vi "pco.camera_Avg_Example_IMAQ.vi"() -> ()   [LabVIEW 2020]
uses:
  Camera.lvclass
panel:
  out "rawImage":u16[][](array[numeric])
  out "Image":T1(plugin-control)
  in  "data_format":T2(ring)=enum."Mono16"
  out "Recorded Images":u32
  in  "Quit":bool
  in  "roiY1":u64=2 min=2 max=1040 step=1
  in  "roiX1":u64=2 min=2 max=1392 step=1
  in  "roiY0":u64=1 min=1 max=1039 step=1
  in  "roiX0":u64=1 min=1 max=1391 step=1
  out "Image Height":u64
  out "Image Width":u64
  in  "dwImgCount":u32=10 caption="Required Number of Images" max=4023
  out "Error":errorcluster {"code" format="%x"}
  # "This example shows how to continously compute and show an averaged image.\nHere the camera class is operated in sequence mode and the required number of images also defines the number of images that will be averaged\nIt is a good starting point for writing own applications.\nBut it will not be fail save, i.e. doesnt react on errors, just handles them forward to the end\n\nUsage:\nSelect your required image count you want to average over before you start the program.\nOnce started, the camera class will be initialized and image record will start automatically.\nInside the acquisition loop the program will record the image sequence.\nThen it calculates the average image and shows it.\nBy using the ROI parameters you can crop the image to select certain regions\n\nBy clicking Quit Application the record will stop and will force an exit of the camera class"
  # "pco.labview"
  # "Camera Setup"
  # "Recording Control"
  # "Parameters for image readout"
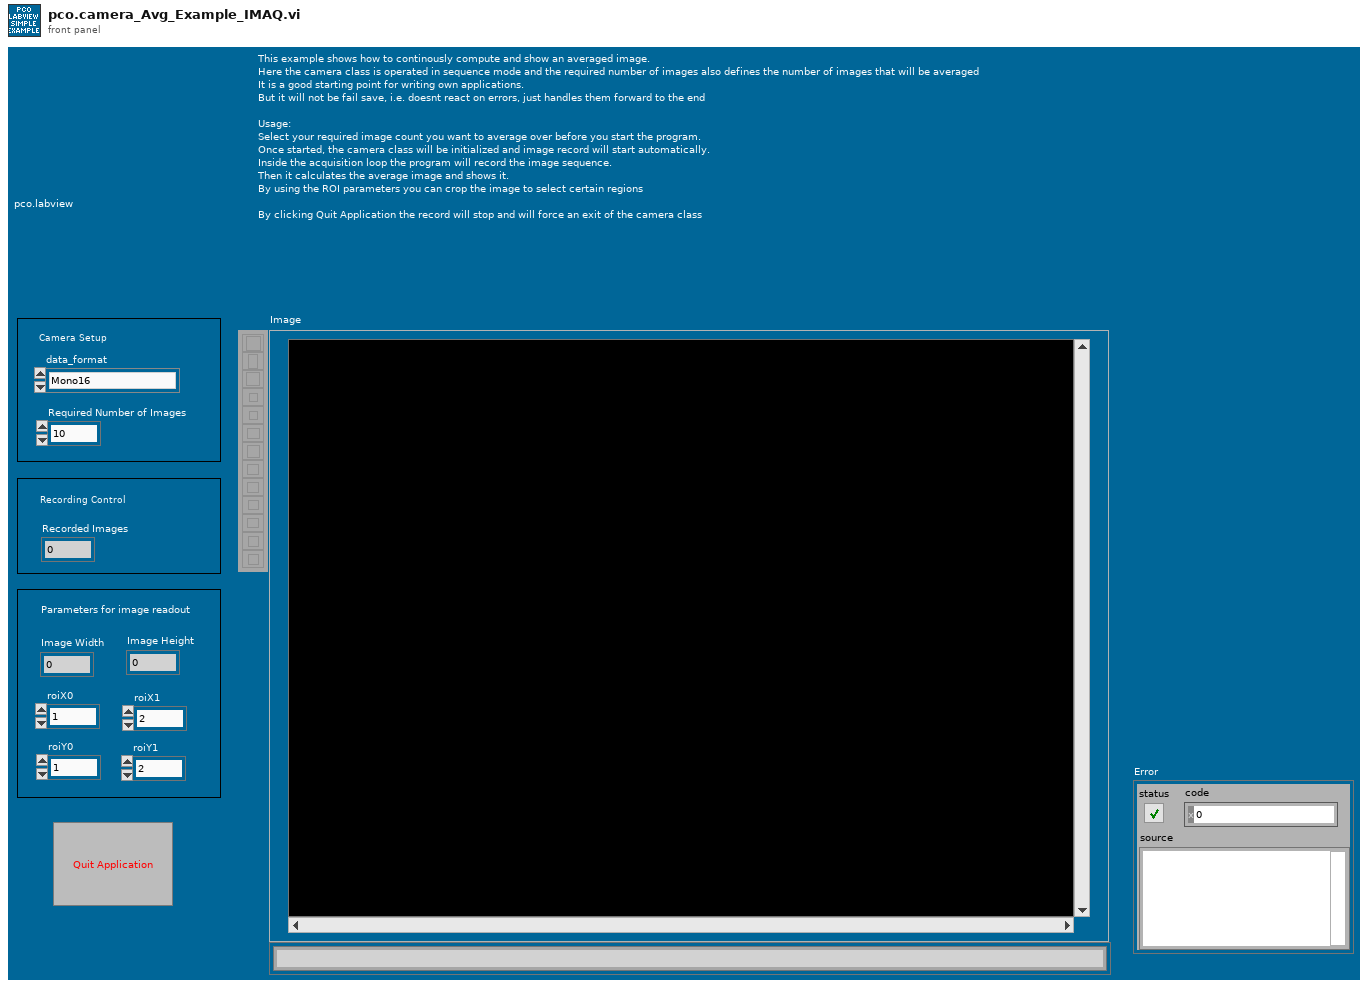
[diagram p1: front panel]
types:
  T1 = typedef "IMAQ Image.ctl" = refnum<image>
  T2 = enum16{"Undefined", "Mono8", "Mono16", "BGRA8", "RGBA8", "BGRA16", "RGBA16", "CompressedMono8"}
  T3 = enum8{"Enabled", "Disabled", "Disabled and Grayed Out"}
  T4 = enum16{"sequence", "sequence non blocking", "ring buffer", "fifo", "sequence_dpcore", "sequence_non_blocking_dpcore", "ring_buffer_dpcore", "fifo_dpcore", "tif", "multitif", "pcoraw", "b16", "dicom", "multidicom"}
  T5 = cluster{"serial":u32, "type":u16, "sub_type":u16, "interface_type":u16, "bit_resolution":u16, "min_exposure_time_s":dbl, "max_exposure_time_s":dbl, "min_exposure_step_s":dbl, "min_delay_time_s":dbl, "max_delay_time_s":dbl, "min_delay_step_s":dbl, "min_width":u64, "min_height":u64, "max_width":u64, "max_height":u64, "roi_step_horz":u64, "roi_step_vert":u64, "roi_symmetric_horz":bool, "roi_symmetric_vert":bool, "has_timestamp_mode":bool, "has_timestamp_mode_ascii_only":bool, "pixelrate_vec":u32[], "has_acquire_mode":bool, "has_ext_acquire_mode":bool, "has_metadata_mode":bool, "has_ram":bool, "binning_horz_vec":u16[], "binning_vert_vec":u16[]}
  T6 = typedef "Image Type" = u32
  T7 = typedef "Camera.lvclass/binning.ctl" = cluster{"vert":u16, "horz":u16}
  T8 = cluster{"exposure_time_s":dbl, "delay_time_s":dbl, "roi":cluster{"x0":u64, "y0":u64, "x1":u64, "y1":u64}, "timestamp_mode":u16, "pixelrate":u32, "trigger_mode":u16, "acquire_mode":u16, "metadata_mode":u16, "noisefilter_mode":u16, "binning":T7}
  T9 = cluster{"Plane 4 (alpha)":u16, "Plane 1 (Red)":u16, "Plane 2 (Green)":u16, "Plane 3 (Blue)":u16}[][]
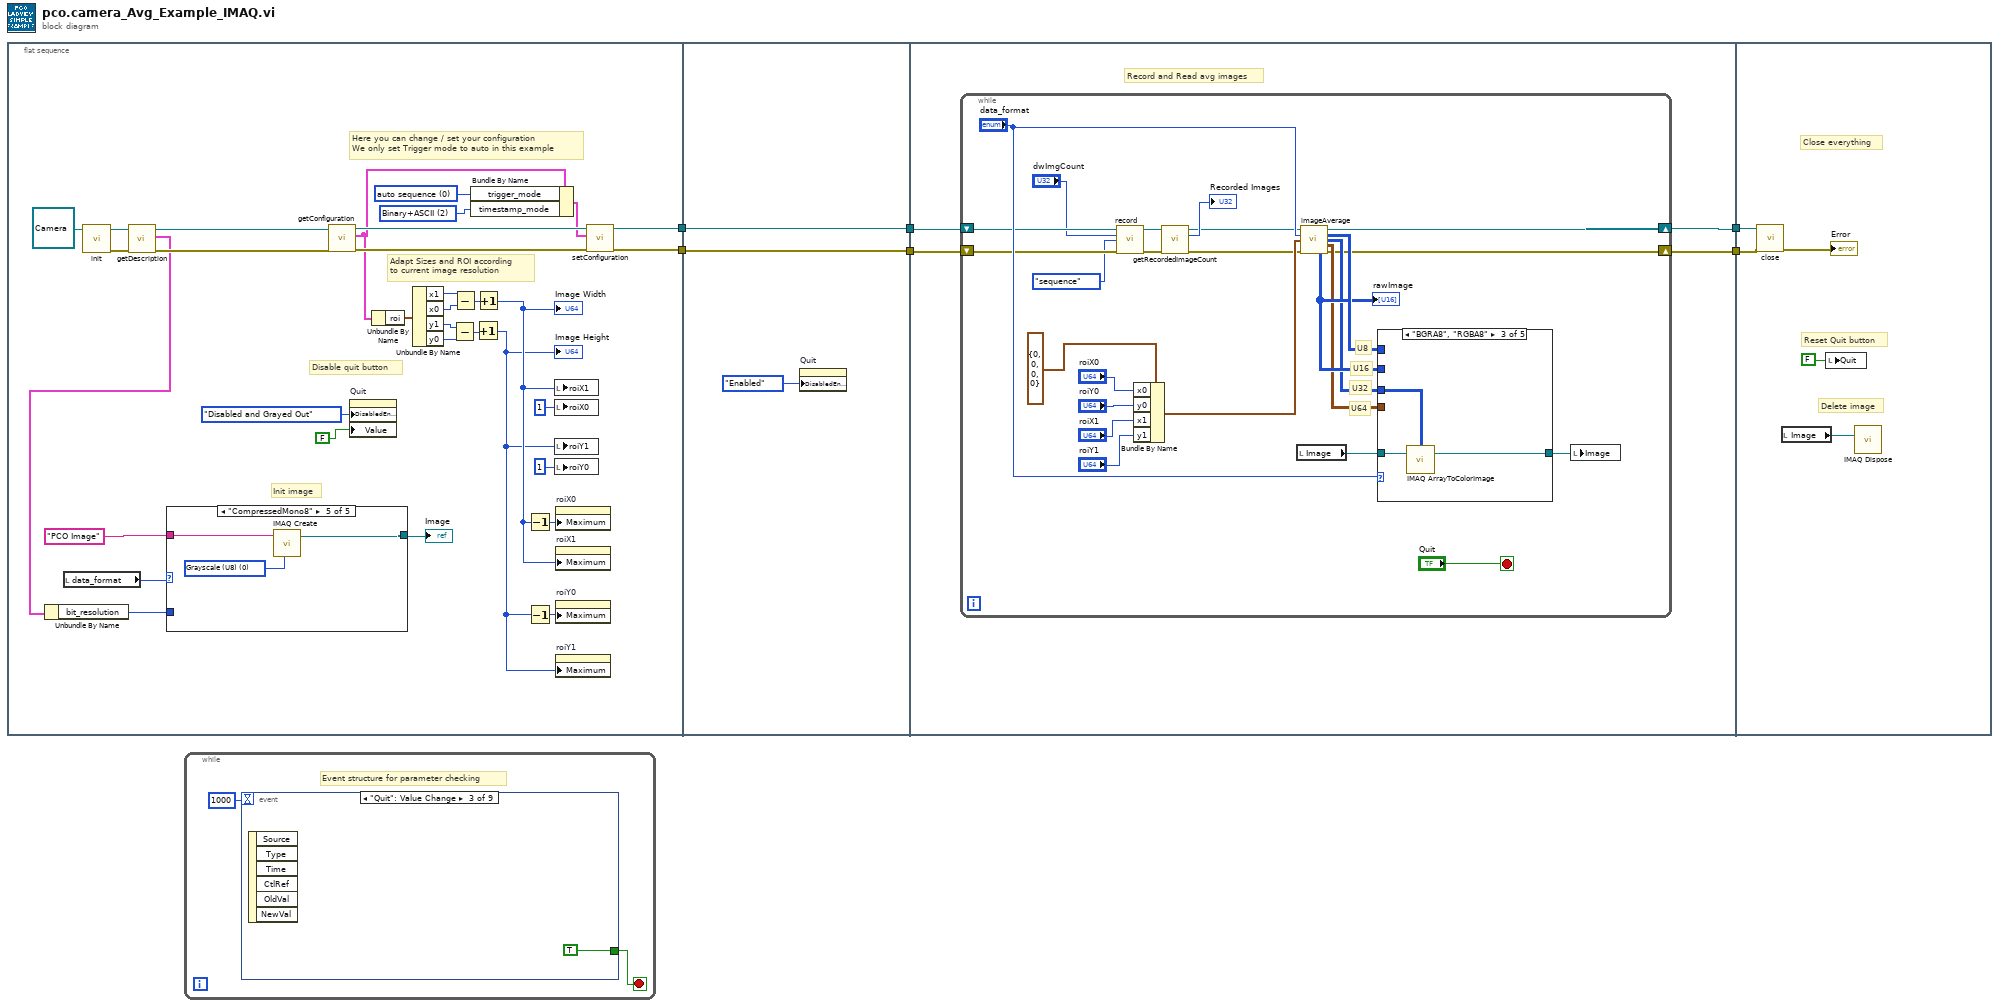
[diagram p0: block diagram]
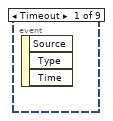
[diagram p2: hidden frame]
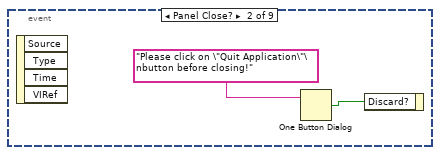
[diagram p3: hidden frame]
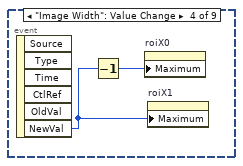
[diagram p4: hidden frame]
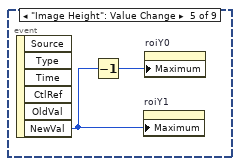
[diagram p5: hidden frame]
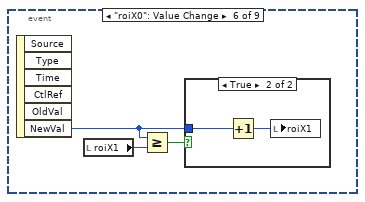
[diagram p6: hidden frame]
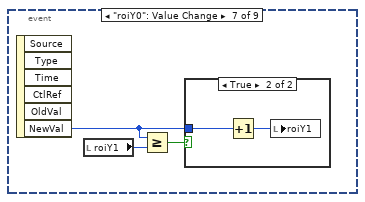
[diagram p8: hidden frame]
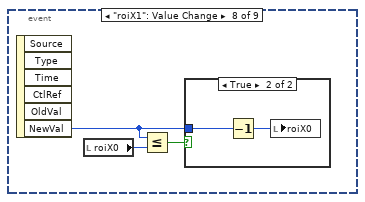
[diagram p10: hidden frame]
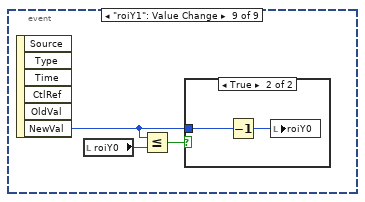
[diagram p12: hidden frame]
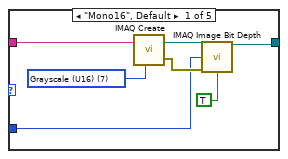
[diagram p14: hidden frame]
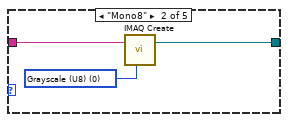
[diagram p15: hidden frame]
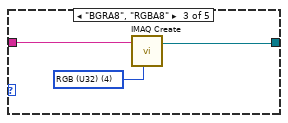
[diagram p16: hidden frame]
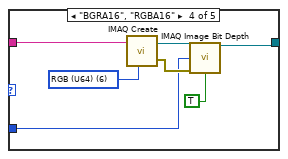
[diagram p17: hidden frame]
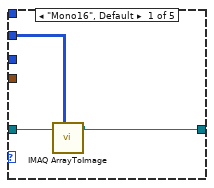
[diagram p18: hidden frame]
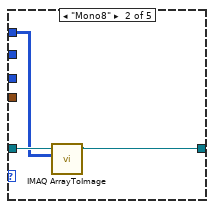
[diagram p19: hidden frame]
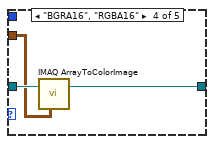
[diagram p20: hidden frame]
diagram:
  n1 = flat-sequence {
    tunnel: [w14] -> w6
    tunnel: [w13] -> w5
    tunnel: w6 -> [w64]
    tunnel: w5 -> [w63]
    tunnel: [w64] -> w4
    tunnel: [w63] -> w3
    tunnel: [w69] -> w2
    tunnel: [w68] -> w1
    tunnel: w3 -> [w67]
    tunnel: w4 -> [w66]
    tunnel: w2 -> [w112]
    tunnel: w1 -> [w111]
    frame #0 {
      w20 = u16 2 items=["OFF", "Binary", "Binary+ASCII", "ASCII"] ("TimestampMode")
      w38 = u16 0 items=["auto sequence"=0, "software trigger"=1, "external exposure start & software trigger"=2, "external exposure control"=3, "external synchronized"=4, "fast external exposure control"=5, "external CDS control"=6, "slow external exposure control"=7, "external synchronized HDSDI"=258] ("TriggerMode")
      # "Init image"
      # "Adapt Sizes and ROI according\nto current image resolution"
      # "Disable quit button"
      # "Here you can change / set your configuration\nWe only set Trigger mode to auto in this example"
      n2 = local read "data_format"() -> (w17:T2)
      n3 = call-dynamic "init.vi"("Camera in"=refnum<class "Camera.lvclass"> refnum ("PCOCamera in")) -> ("Camera out"=w11:refnum<class "Camera.lvclass">, "error out"=w12:errorcluster)  [unwired: 8 in]
      n4 = call-dynamic "getDescription.vi"("error in (no error)"=w12, "Camera in"=w11) -> ("error out"=w9:errorcluster, "description"=w8:T5, "Camera out"=w10:refnum<class "Camera.lvclass">)  [unwired: 7 in]
      n5 = Unbundle By Name(w8) -> ("bit_resolution"=w7:u16)
      n6 = case shown="\"CompressedMono8\"" w17 {
        tunnel: "PCO Image" ("Image Name") -> [w45 w49 w51 w58 w61]
        tunnel: [w41 w47 w50 w54 w60] -> w16
        tunnel: w7 -> [w40 _ _ w53 _]
        frame "Mono16", Default {
          w46 = T6 7 items=["Grayscale (U8)", "Grayscale (I16)", "Grayscale (SGL)", "Complex (CSG)", "RGB (U32)", "HSL (U32)", "RGB (U64)", "Grayscale (U16)"] ("Image Type")
          n7 = call "IMAQ Create"("Image Name"=w45, "Image Type"=w46) -> ("New Image"=w43:T1, "error out"=w42:errorcluster)  [unwired: 3 in]
          n8 = call "IMAQ Image Bit Depth"("Image"=w43, "Bit Depth (0)"=w40, "error in (no error)"=w42, "Get/Set Bit Depth? (Set)"=TRUE) -> ("Image Out"=w41:T1)  [unwired: 9 in, 2 out]
        }
        frame "Mono8" {
          w48 = T6 0 items=["Grayscale (U8)", "Grayscale (I16)", "Grayscale (SGL)", "Complex (CSG)", "RGB (U32)", "HSL (U32)", "RGB (U64)", "Grayscale (U16)"] ("Image Type")
          n9 = call "IMAQ Create"("Image Name"=w49, "Image Type"=w48) -> ("New Image"=w47:T1)  [unwired: 3 in, 1 out]
        }
        frame "BGRA8", "RGBA8" {
          w52 = T6 4 items=["Grayscale (U8)", "Grayscale (I16)", "Grayscale (SGL)", "Complex (CSG)", "RGB (U32)", "HSL (U32)", "RGB (U64)", "Grayscale (U16)"] ("Image Type")
          n10 = call "IMAQ Create"("Image Name"=w51, "Image Type"=w52) -> ("New Image"=w50:T1)  [unwired: 3 in, 1 out]
        }
        frame "BGRA16", "RGBA16" {
          w59 = T6 6 items=["Grayscale (U8)", "Grayscale (I16)", "Grayscale (SGL)", "Complex (CSG)", "RGB (U32)", "HSL (U32)", "RGB (U64)", "Grayscale (U16)"] ("Image Type")
          n11 = call "IMAQ Create"("Image Name"=w58, "Image Type"=w59) -> ("New Image"=w56:T1, "error out"=w55:errorcluster)  [unwired: 3 in]
          n12 = call "IMAQ Image Bit Depth"("Image"=w56, "Bit Depth (0)"=w53, "error in (no error)"=w55, "Get/Set Bit Depth? (Set)"=TRUE) -> ("Image Out"=w54:T1)  [unwired: 9 in, 2 out]
        }
        frame "CompressedMono8" {
          w62 = T6 0 items=["Grayscale (U8)", "Grayscale (I16)", "Grayscale (SGL)", "Complex (CSG)", "RGB (U32)", "HSL (U32)", "RGB (U64)", "Grayscale (U16)"] ("Image Type")
          n13 = call "IMAQ Create"("Image Name"=w61, "Image Type"=w62) -> ("New Image"=w60:T1)  [unwired: 3 in, 1 out]
        }
      }
      "Image" <- w16
      n14 = call-dynamic "getConfiguration.vi"("error in (no error)"=w9, "Camera in"=w10) -> ("error out"=w36:errorcluster, "configuration"=w30:T8, "Camera out"=w37:refnum<class "Camera.lvclass">)  [unwired: 7 in]
      n15 = property on="Quit" class="Bool (strict)"("DisabledEnum"=T3."Disabled and Grayed Out" ("Disabled"), "Value"=FALSE ("Stop")) -> ()  [unwired: 2 in, 2 out]
      n16 = Unbundle By Name(w30) -> ("roi"=w29:cluster{"x0":u64, "y0":u64, "x1":u64, "y1":u64})
      n17 = Unbundle By Name(w29) -> ("x1"=w27:u64, "x0"=w28:u64, "y1"=w25:u64, "y0"=w26:u64)
      n18 = Subtract(x=w25, y=w26) -> (x-y=w23:u64)
      n19 = Subtract(x=w27, y=w28) -> (x-y=w24:u64)
      n20 = Bundle By Name(cluster=w30, "trigger_mode"=w38, "timestamp_mode"=w20) -> (w35:T8)
      n21 = Increment(x=w23) -> (x+1=w21:u64)
      "Image Height" <- w21
      n22 = Increment(x=w24) -> (x+1=w22:u64)
      "Image Width" <- w22
      n23 = Decrement(x=w22) -> (x-1=w32:u64)
      n24 = Decrement(x=w21) -> (x-1=w31:u64)
      n25 = local write "roiX1"(w22) -> ()
      n26 = local write "roiX0"(u64 1 ("roiY0")) -> ()
      n27 = local write "roiY1"(w21) -> ()
      n28 = local write "roiY0"(u64 1 ("roiY0")) -> ()
      n29 = property on="roiX0" class="DigNum (strict)"("Maximum"=w32) -> ()  [unwired: 2 in, 2 out]
      n30 = property on="roiX1" class="DigNum (strict)"("Maximum"=w22) -> ()  [unwired: 2 in, 2 out]
      n31 = property on="roiY0" class="DigNum (strict)"("Maximum"=w31) -> ()  [unwired: 2 in, 2 out]
      n32 = property on="roiY1" class="DigNum (strict)"("Maximum"=w21) -> ()  [unwired: 2 in, 2 out]
      n33 = call-dynamic "setConfiguration.vi"("error in (no error)"=w36, "configuration"=w35, "Camera in"=w37) -> ("error out"=w13:errorcluster, "Camera out"=w14:refnum<class "Camera.lvclass">)  [unwired: 7 in]
    }
    frame #1 {
      n34 = property on="Quit" class="Bool (strict)"("DisabledEnum"=T3."Enabled" ("Disabled")) -> ()  [unwired: 2 in, 2 out]
    }
    frame #2 {
      # "Record and Read avg images"
      n35 = while {
        shift-right: [w80] -> w69
        shift-left: w66 -> [w79]
        shift-right: [w70] -> w68
        shift-left: w67 -> [w78]
        stop <- "Quit" stop-if-true
        # "U64"
        # "U32"
        # "U16"
        # "U8"
        n36 = call-dynamic "record.vi"("Camera in"=w79, "num_images"="dwImgCount", "record_mode"=T4."sequence", "error in (no error)"=w78) -> ("Camera out"=w76:refnum<class "Camera.lvclass">, "error out"=w75:errorcluster)  [unwired: 10 in]
        n37 = Bundle By Name(cluster=cluster{"x0":u64, "y0":u64, "x1":u64, "y1":u64} {"x0"=0, "y0"=0, "x1"=0, "y1"=0} ("roi"), "x0"="roiX0", "y0"="roiY0", "x1"="roiX1", "y1"="roiY1") -> (w90:cluster{"x0":u64, "y0":u64, "x1":u64, "y1":u64})
        n38 = call-dynamic "getRecordedImageCount.vi"("Camera in"=w76, "error in (no error)"=w75) -> ("Camera out"=w73:refnum<class "Camera.lvclass">, "recorded_image_count"=→"Recorded Images":u32, "error out"=w72:errorcluster)  [unwired: 11 in]
        n39 = local read "Image"() -> (w84:T1)
        n40 = call-dynamic "imageAverage.vi"("Camera in"=w73, "data_format"="data_format", "roi"=w90, "error in (no error)"=w72) -> ("Camera out"=w80:refnum<class "Camera.lvclass">, "image (U8)"=w88:u8[][], "image (U32)"=w86:u32[][], "image (U64)"=w85:T9, "raw_image (U16)"=w87:u16[][], "error out"=w70:errorcluster)  [unwired: 6 in]
        "rawImage" <- w87
        n41 = case shown="\"BGRA8\", \"RGBA8\"" "data_format" {
          tunnel: w84 -> [w97 w100 w103 w106 w109]
          tunnel: [w95 w98 w102 w104 w108] -> w83
          tunnel: w85 -> [_ _ _ w105 _]
          tunnel: w86 -> [_ _ w101 _ _]
          tunnel: w88 -> [_ w99 _ _ w107]
          tunnel: w87 -> [w96 _ _ _ _]
          frame "Mono16", Default {
            n42 = call "IMAQ ArrayToImage"("Image Pixels (U16)"=w96, "Image"=w97) -> ("Image Out"=w95:T1)  [unwired: 8 in, 1 out]
          }
          frame "Mono8" {
            n43 = call "IMAQ ArrayToImage"("Image Pixels (U8)"=w99, "Image"=w100) -> ("Image Out"=w98:T1)  [unwired: 8 in, 1 out]
          }
          frame "BGRA8", "RGBA8" {
            n44 = call "IMAQ ArrayToColorImage"("Image Pixels (U32)"=w101, "Image"=w103) -> ("Image Out"=w102:T1)  [unwired: 3 in, 1 out]
          }
          frame "BGRA16", "RGBA16" {
            n45 = call "IMAQ ArrayToColorImage"("Image"=w106, "Image Pixels (U64)"=w105) -> ("Image Out"=w104:T1)  [unwired: 3 in, 1 out]
          }
          frame "CompressedMono8" {
            n46 = call "IMAQ ArrayToImage"("Image Pixels (U8)"=w107, "Image"=w109) -> ("Image Out"=w108:T1)  [unwired: 8 in, 1 out]
          }
        }
        n47 = local write "Image"(w83) -> ()
      }
    }
    frame #3 {
      # "Delete image"
      # "Reset Quit button"
      # "Close everything"
      n48 = call-dynamic "close.vi"("error in (no error)"=w111, "Camera in"=w112) -> ("error out"=→"Error":errorcluster)  [unwired: 9 in]
      n49 = local read "Image"() -> (w110:T1)
      n50 = local write "Quit"(FALSE ("Stop")) -> ()
      n51 = call "IMAQ Dispose"("Image"=w110) -> ()  [unwired: 5 in, 1 out]
    }
  }
  n52 = while {
    stop <- w115 stop-if-true
    # "Event structure for parameter checking"
    n53 = event shown="[2] \"Quit\": Value Change" {
      selector: _ -> [_ _ _ _ _ _ _ _ _]
      dyn-events: _ -> [_ _ _ _ _ _ _ _ _]
      timeout: 1000 -> [_ _ _ _ _ _ _ _ _]
      tunnel: [_ _ TRUE _ _ _ _ _ _] -> w115
      event Timeout {
        n54 = event-data() -> ()  [unwired: 1 in, 3 out]
      }
      event Panel Close? {
        n55 = event-data() -> ()  [unwired: 1 in, 4 out]
        n56 = One Button Dialog(message="Please click on \"Quit Application\"\nbutton before closing!") -> (true=w117:bool)  [unwired: 1 in]
        n57 = event-data("Discard?"=w117) -> ()  [unwired: 1 in, 1 out]
      }
      event "Quit": Value Change {
        n58 = event-data() -> ()  [unwired: 1 in, 6 out]
      }
      event "Image Width": Value Change {
        n59 = event-data() -> ("NewVal"=w120:u64)  [unwired: 1 in, 5 out]
        n60 = Decrement(x=w120) -> (x-1=w121:u64)
        n61 = property on="roiX0" class="DigNum (strict)"("Maximum"=w121) -> ()  [unwired: 2 in, 2 out]
        n62 = property on="roiX1" class="DigNum (strict)"("Maximum"=w120) -> ()  [unwired: 2 in, 2 out]
      }
      event "Image Height": Value Change {
        n63 = event-data() -> ("NewVal"=w122:u64)  [unwired: 1 in, 5 out]
        n64 = Decrement(x=w122) -> (x-1=w123:u64)
        n65 = property on="roiY1" class="DigNum (strict)"("Maximum"=w122) -> ()  [unwired: 2 in, 2 out]
        n66 = property on="roiY0" class="DigNum (strict)"("Maximum"=w123) -> ()  [unwired: 2 in, 2 out]
      }
      event "roiX0": Value Change {
        n67 = event-data() -> ("NewVal"=w124:u64)  [unwired: 1 in, 5 out]
        n68 = local read "roiX1"() -> (w126:u64)
        n69 = Greater Or Equal?(x=w124, y=w126) -> (x >= y?=w125:bool)
        n70 = case shown="True" w125 {
          tunnel: w124 -> [_ w128]
          frame False {
          }
          frame True {
            n71 = Increment(x=w128) -> (x+1=w127:u64)
            n72 = local write "roiX1"(w127) -> ()
          }
        }
      }
      event "roiY0": Value Change {
        n73 = event-data() -> ("NewVal"=w129:u64)  [unwired: 1 in, 5 out]
        n74 = local read "roiY1"() -> (w131:u64)
        n75 = Greater Or Equal?(x=w129, y=w131) -> (x >= y?=w130:bool)
        n76 = case shown="True" w130 {
          tunnel: w129 -> [_ w133]
          frame False {
          }
          frame True {
            n77 = Increment(x=w133) -> (x+1=w132:u64)
            n78 = local write "roiY1"(w132) -> ()
          }
        }
      }
      event "roiX1": Value Change {
        n79 = event-data() -> ("NewVal"=w134:u64)  [unwired: 1 in, 5 out]
        n80 = local read "roiX0"() -> (w136:u64)
        n81 = Less Or Equal?(x=w134, y=w136) -> (x <= y?=w135:bool)
        n82 = case shown="True" w135 {
          tunnel: w134 -> [_ w138]
          frame False {
          }
          frame True {
            n83 = Decrement(x=w138) -> (x-1=w137:u64)
            n84 = local write "roiX0"(w137) -> ()
          }
        }
      }
      event "roiY1": Value Change {
        n85 = event-data() -> ("NewVal"=w139:u64)  [unwired: 1 in, 5 out]
        n86 = local read "roiY0"() -> (w141:u64)
        n87 = Less Or Equal?(x=w139, y=w141) -> (x <= y?=w140:bool)
        n88 = case shown="True" w140 {
          tunnel: w139 -> [_ w143]
          frame False {
          }
          frame True {
            n89 = Decrement(x=w143) -> (x-1=w142:u64)
            n90 = local write "roiY0"(w142) -> ()
          }
        }
      }
    }
  }
